vi "check_and_correct_input.vi"(4 "delay array":dbl[](array[numeric])) -> (1 "corrrected delay array":dbl[](array[numeric]))   [LabVIEW 2011]
doc: "Check if all the values entered by the user are correct. See the block diagram for the rules and add some if need be. \nThis vi also makes noise and shows the user what he did wrong!"
panel:
  # "check for correct data entry, \ncorrect data if necessary,\n play sound if input was wrong \nand show what was wrong"
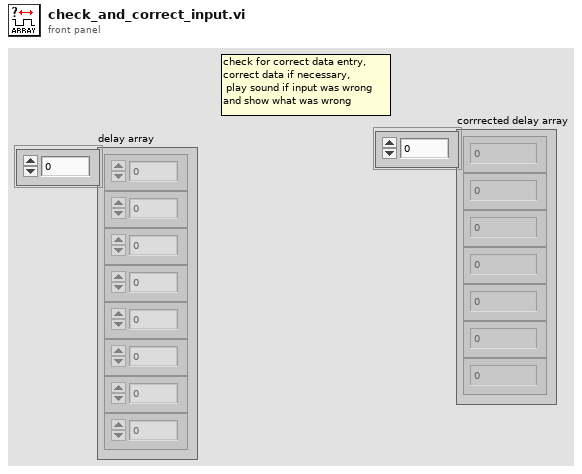
[diagram p1: front panel]
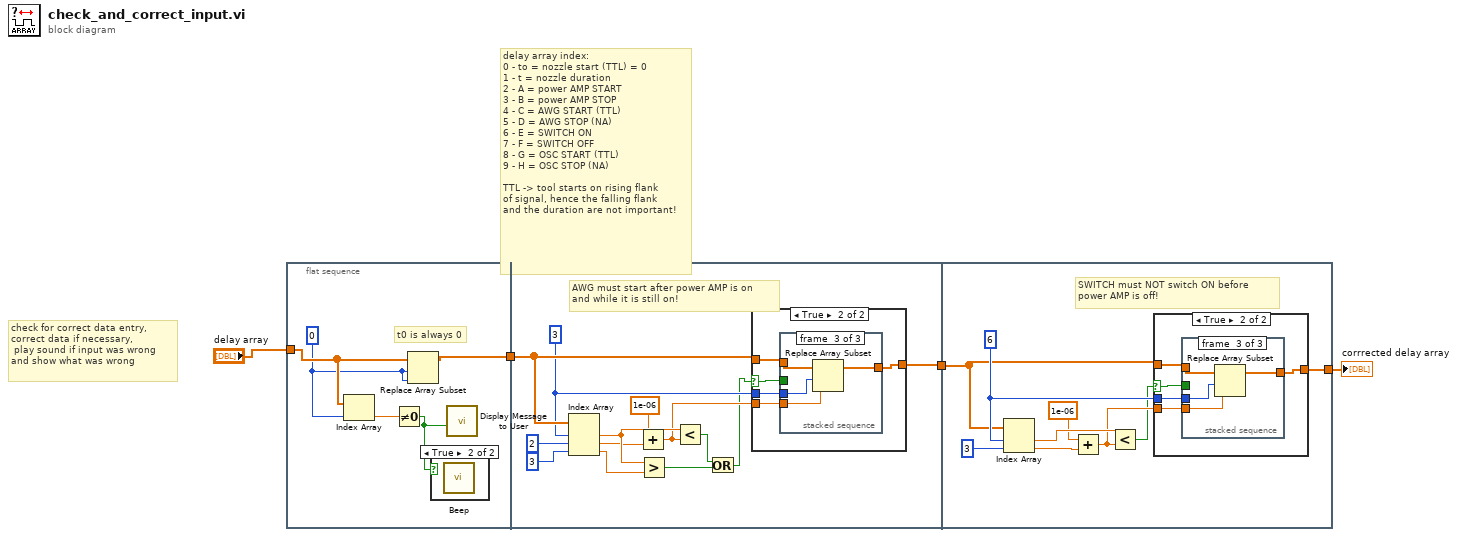
[diagram p0: block diagram]
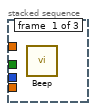
[diagram p4: hidden frame]
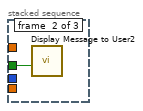
[diagram p5: hidden frame]
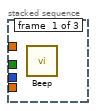
[diagram p7: hidden frame]
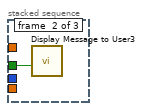
[diagram p8: hidden frame]
diagram:
  # "check for correct data entry, \ncorrect data if necessary,\n play sound if input was wrong \nand show what was wrong"
  # "delay array index:\n0 - to = nozzle start (TTL) = 0\n1 - t = nozzle duration\n2 - A = power AMP START\n3 - B = power AMP STOP\n4 - C = AWG START (TTL)\n5 - D = AWG STOP (NA)\n6 - E = SWITCH ON \n7 - F = SWITCH OFF\n8 - G = OSC START (TTL)\n9 - H = OSC STOP (NA)\n\nTTL -> tool starts on rising flank\nof signal, hence the falling flank \nand the duration are not important!"
  n1 = flat-sequence {
    tunnel: "delay array" -> [w9]
    tunnel: [w8] -> w3
    tunnel: w3 -> [w16]
    tunnel: [w10] -> w2
    tunnel: w2 -> [w37]
    tunnel: [w34] -> w1
    frame #0 {
      w6 = 0 ("index")
      # "t0 is always 0"
      n2 = Index Array(array=w9, index=w6) -> (element=w5:dbl)
      n3 = Not Equal To 0?(x=w5) -> (x != 0?=w7:bool)
      n4 = Replace Array Subset(array=w9, new element=w6, index=w6) -> (w8:dbl[])
      n5 = case shown="True" w7 {
        frame False {
        }
        frame True {
          n6 = call <vilib>:"Beep.vi"() -> ()  [unwired: 12 in]
        }
      }
      n7 = call "Display Message to User"("Enable"=w7) -> ()  [unwired: 9 in, 2 out]
    }
    frame #1 {
      w14 = 3 ("index")
      # "AWG must start after power AMP is on \nand while it is still on!"
      n8 = Index Array(array=w16, index #1=w14, index #2=2 ("index"), index #3=3 ("index")) -> (element #1=w20:dbl, element #2=w18:dbl, element #3=w19:dbl)
      n9 = Add(x=1e-06, y=w18) -> (x+y=w13:dbl)
      n10 = Greater?(x=w20, y=w19) -> (0:w15:bool)
      n11 = Less?(x=w20, y=w13) -> (x < y?=w11:bool)
      n12 = Or(x=w11, y=w15) -> (x .or. y?=w12:bool)
      n13 = case shown="True" w12 {
        selector: w12 -> [_ w28]
        tunnel: [w23 w27] -> w10
        tunnel: w16 -> [w23 w26]
        tunnel: w14 -> [_ w25]
        tunnel: w13 -> [_ w24]
        frame False {
        }
        frame True {
          n14 = stacked-sequence {
            tunnel: w28 -> [_ w29 _]
            tunnel: [_ _ w33] -> w27
            tunnel: w26 -> [_ _ w32]
            tunnel: w25 -> [_ _ w31]
            tunnel: w24 -> [_ _ w30]
            frame #0 {
              n15 = call <vilib>:"Beep.vi"() -> ()  [unwired: 12 in]
            }
            frame #1 {
              n16 = call "Display Message to User2"("Enable"=w29) -> ()  [unwired: 9 in, 2 out]
            }
            frame #2 {
              n17 = Replace Array Subset(array=w32, new element=w30, index=w31) -> (w33:dbl[])
            }
          }
        }
      }
    }
    frame #2 {
      w39 = 6 ("index")
      # "SWITCH must NOT switch ON before \npower AMP is off!"
      n18 = Index Array(array=w37, index #1=w39, index #2=3 ("index")) -> (element #1=w41:dbl, element #2=w35:dbl)
      n19 = Add(x=1e-06, y=w35) -> (x+y=w38:dbl)
      n20 = Less?(x=w41, y=w38) -> (x < y?=w36:bool)
      n21 = case shown="True" w36 {
        selector: w36 -> [_ w48]
        tunnel: [w43 w47] -> w34
        tunnel: w37 -> [w43 w46]
        tunnel: w39 -> [_ w45]
        tunnel: w38 -> [_ w44]
        frame False {
        }
        frame True {
          n22 = stacked-sequence {
            tunnel: w48 -> [_ w49 _]
            tunnel: [_ _ w53] -> w47
            tunnel: w46 -> [_ _ w52]
            tunnel: w45 -> [_ _ w51]
            tunnel: w44 -> [_ _ w50]
            frame #0 {
              n23 = call <vilib>:"Beep.vi"() -> ()  [unwired: 12 in]
            }
            frame #1 {
              n24 = call "Display Message to User3"("Enable"=w49) -> ()  [unwired: 9 in, 2 out]
            }
            frame #2 {
              n25 = Replace Array Subset(array=w52, new element=w50, index=w51) -> (w53:dbl[])
            }
          }
        }
      }
    }
  }
  "corrrected delay array" <- w1
